vi "MakeRadialAxis (SubVI).vi"(1 "# radial bins":u32, 2 "Rmin":dbl, 3 "Rmax-Rmin":dbl) -> (0 "radialaxis":dbl[](array[numeric]))   [LabVIEW 2011, in "OfflineTracker.lvlib"]
uses:
  OfflineTracker.lvlib
panel:
  out "Waveform Graph":dbl[](graph)
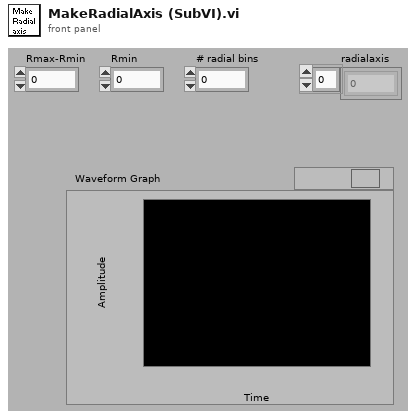
[diagram p1: front panel]
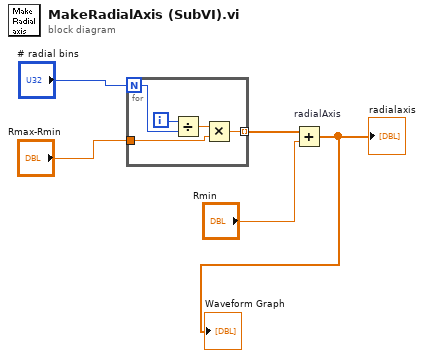
[diagram p0: block diagram]
diagram:
  n1 = for {
    N: "# radial bins" -> [w9]
    tunnel: "Rmax-Rmin" -> [w8]
    tunnel: [w6] -> w2 mode=indexing
    i -> [w10]
    n2 = Divide(x=w10, y=w9) -> (x/y=w7:dbl)
    n3 = Multiply(x=w7, y=w8) -> (x*y=w6:dbl)
  }
  n4 = Add "radialAxis"(x=w2, y="Rmin") -> (x+y=→"radialaxis" →"Waveform Graph":dbl[])
